vi "K2602A_SetCurrent.vi"(0 "VISA resource name":refnum<visa-resource-name>="GPIB0::26::INSTR", 1 "Channel (1or2)":dbl, 2 "Set Current (A)":dbl, 3 "error in (no error)":errorcluster, 4 "Range (A)":dbl=0.001) -> (5 "error out":T1)   [LabVIEW 2014]
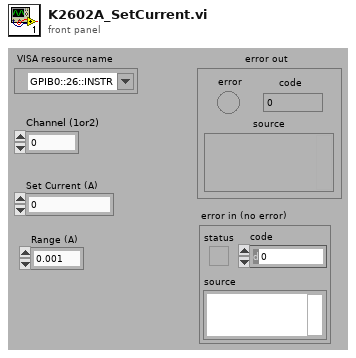
[diagram p1: front panel]
types:
  T1 = cluster{"error":bool, "code":i32, "source":string}
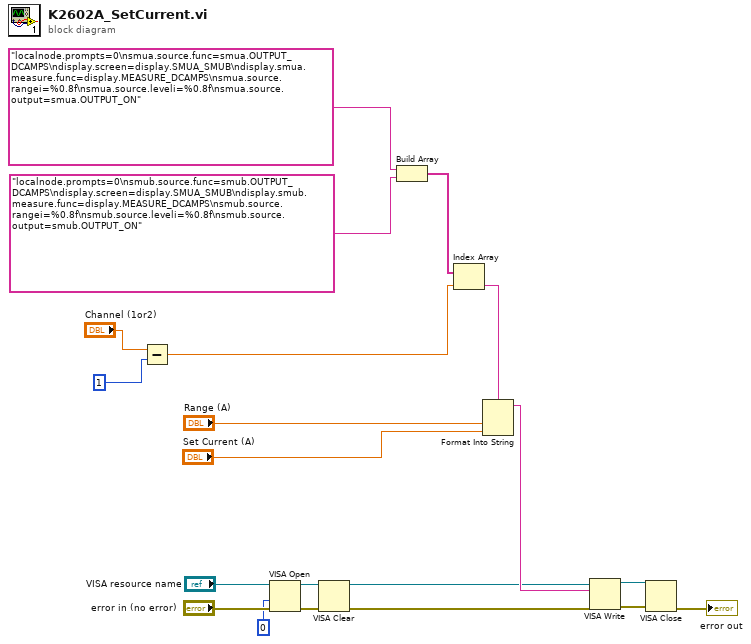
[diagram p0: block diagram]
diagram:
  n1 = Subtract(x="Channel (1or2)", y=u32 1 ("access mode")) -> (x-y=w20:dbl)
  n2 = VISA Open(access mode=u32 0, error in (no error)="error in (no error)", VISA resource name="VISA resource name") -> (VISA resource name=w2:refnum<visa-resource-name>, error out=w3:errorcluster)  [unwired: 2 out]
  n3 = VISA Clear(VISA resource name=w2, error in (no error)=w3) -> (VISA resource name out=w6:refnum<visa-resource-name>, error out=w7:errorcluster)
  n4 = Build Array("localnode.prompts=0\nsmua.source.func=smua.OUTPUT_DCAMPS\ndisplay.screen=display.SMUA_SMUB\ndisplay.smua.measure.func=display.MEASURE_DCAMPS\nsmua.source.rangei=%0.8f\nsmua.source.leveli=%0.8f\nsmua.source.output=smua.OUTPUT_ON", "localnode.prompts=0\nsmub.source.func=smub.OUTPUT_DCAMPS\ndisplay.screen=display.SMUA_SMUB\ndisplay.smub.measure.func=display.MEASURE_DCAMPS\nsmub.source.rangei=%0.8f\nsmub.source.leveli=%0.8f\nsmub.source.output=smub.OUTPUT_ON") -> (w16:string[])
  n5 = Index Array(array=w16, index=w20) -> (element=w17:string)
  n6 = Format Into String(format string=w17, "Range (A)", "Set Current (A)") -> (resulting string=w11:string)  [unwired: 2 in, 1 out]
  n7 = VISA Write(VISA resource name=w6, write buffer=w11, error in (no error)=w7) -> (VISA resource name out=w8:refnum<visa-resource-name>, error out=w9:errorcluster)  [unwired: 1 out]
  n8 = VISA Close(VISA resource name=w8, error in (no error)=w9) -> (error out=→"error out":errorcluster)
